vi "Control UI - Gain and Offset Exploration.vi"(9 "Active DUT index":i32 min=0 max=3 step=1, 10 "ESR scaling ref":refnum<vi>, 11 "Main Ref":refnum<class "Main.lvclass">) -> ()   [LabVIEW 2019, in "Main.lvclass"]
doc: "Developed by Kevin Thompson\nkevin@thompsonengineering.net\n\nCopyright 2020\nThompson Engineering, LLC"
uses:
  Main.lvclass
  support/Data Algorithms/subvis/DataTypes/ESR scaling--cluster.ctl
  Common/DataTypes/Inverter database record v2--cluster.ctl
  Common/DataTypes/inverter info v2--cluster.ctl
  Common/DataTypes/inverter gain range--cluster.ctl
  Common/DataTypes/inverter offset range--cluster.ctl
  Main.lvclass/Main.ctl
panel:
  in  "Direction":bool caption="Auto Increment Direction"
  in  "SetOffsetToMax":bool
  in  "SetGainToMax":bool
  in  "SetOffsetToMin":bool
  in  "SetGainToMin":bool
  in  "ResetGainOffsetRng":bool caption="Reset Gain/Offset\nRanges"
  in  "Exit":bool
  in  "Scaling Sel":enum32{"select gain", "select offset"}(radio) caption="Scaling Selection"
  in  "AutoIncrIntv (sec)":dbl(slide)=2.0 caption="Auto Increment Interval (sec)" min=2.0 max=20.0 step=1.0 scale=2.0..20.0
  out "AutoIncr LED":bool caption="Auto Incrementing"
  in  "StopAutoIncr":bool
  in  "StartAutoIncr":bool
  in  "offset range":T1
  in  "gain range":T2
  out "name":string caption="Inverter Name"
  out "CurrInverter":T3 {"last updated" format="%<%H:%M\n%d/%m/%Y>T"; "set flag" items=["False", "True"]}
  in  "StepBack":bool
  in  "StepFwd":bool
  in  "ESR scaling":T5={"Gain"=1.0, "Offset"=0.0} caption="Current ESR scaling" {"Offset" format="%^#_6g"; "Gain" format="%^#_6g"}
  # "Direction"
  # "increasing"
  # "decreasing"
  # "Inverter Gain & Offset Setting Explorer"
  # "Inverter Offset Range"
  # "Inverter Gain Range"
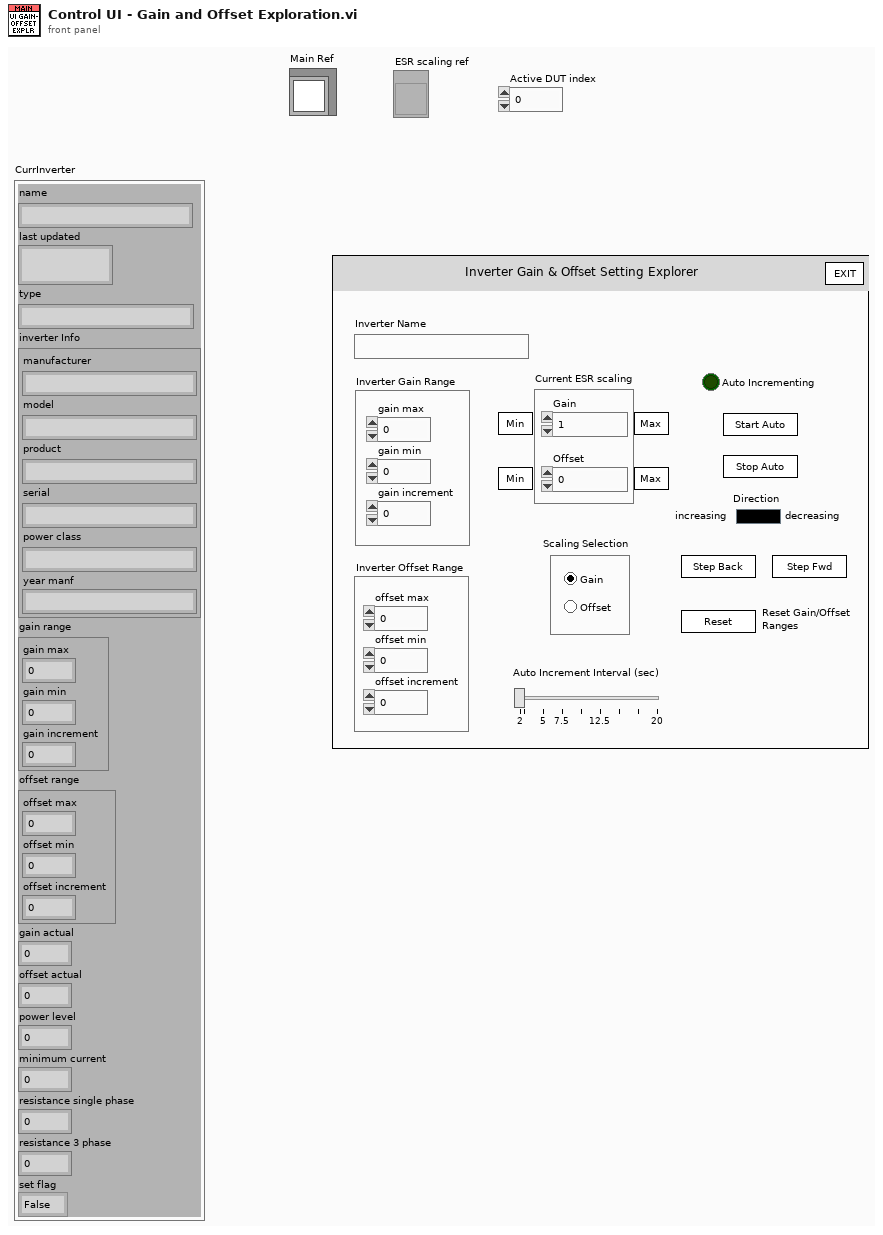
[diagram p1: front panel]
types:
  T1 = typedef "inverter offset range--cluster.ctl" = cluster{"offset max":dbl, "offset min":dbl, "offset increment":dbl}
  T2 = typedef "inverter gain range--cluster.ctl" = cluster{"gain max":dbl, "gain min":dbl, "gain increment":dbl}
  T3 = typedef "Inverter database record v2--cluster.ctl" = cluster{"name":string, "last updated":timestamp, "type":string, "inverter Info":T4, "gain range":T2, "offset range":T1, "gain actual":dbl, "offset actual":dbl, "power level":dbl, "minimum current":dbl, "resistance single phase":dbl, "resistance 3 phase":dbl, "set flag":u16}
  T4 = typedef "inverter info v2--cluster.ctl" = cluster{"manufacturer":string, "model":string, "product":string, "serial":string, "power class":string, "year manf":string}
  T5 = typedef "Main.lvclass/ESR scaling--cluster.ctl" = cluster{"Gain":dbl, "Offset":dbl}
  T6 = enum32{"invalid app kind", "Development System", "Run Time System", "Student Edition", "Embedded LabVIEW", "Evaluation", "Custom"}
  T7 = enum32{"Invalid", "Standard", "Closed", "Hidden", "Minimized", "Maximized"}
  T8 = cluster{"Main out":refnum<class "Main.lvclass">, "Core":cluster{"Current VI Reference":refnum<vi>, "Close Panel on Exit?":bool}, "ESR scaling ref":refnum<vi>, "ESR scaling":T5, "AutoIncr Enabled":bool, "Scaling Sel":enum32{"select gain", "select offset"}, "AutoIncrIntv (sec)":dbl, "ESR scaling - UI Label":string, "CurrInverter":T3, "gain range":T2, "offset range":T1, "Direction":bool, "LimitReached":bool}
  T9 = cluster{"Current VI Reference":refnum<vi>, "Close Panel on Exit?":bool}
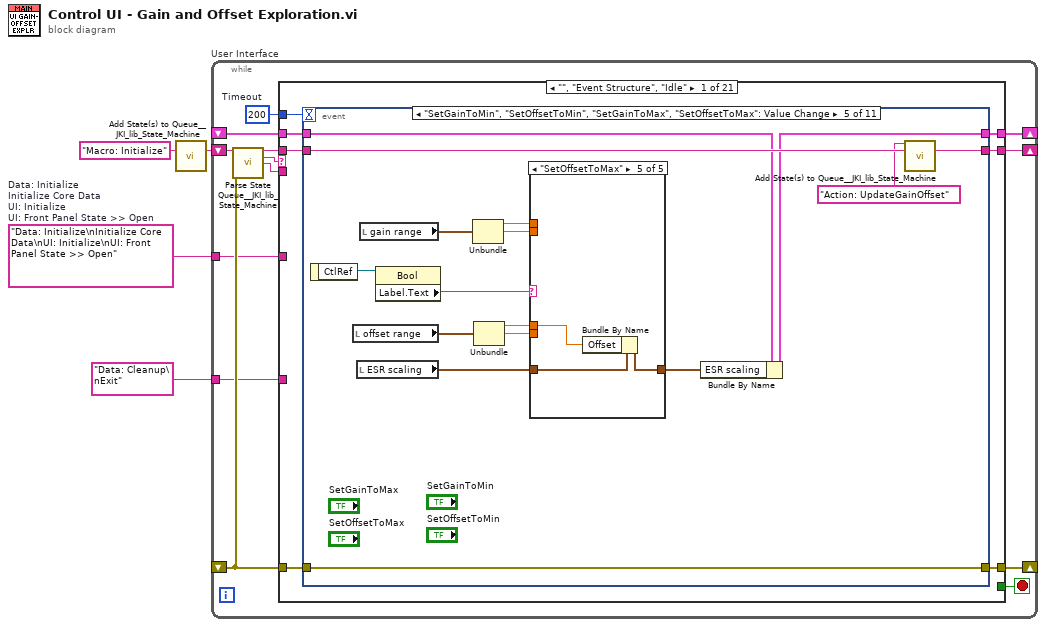
[diagram p0: block diagram]
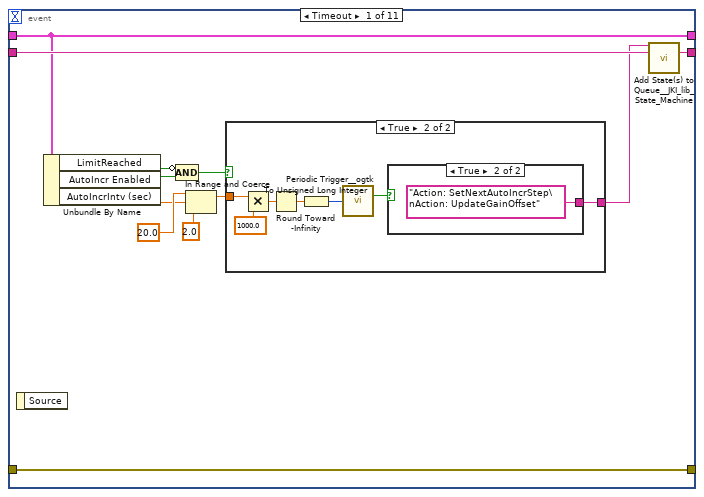
[diagram p2: hidden frame]
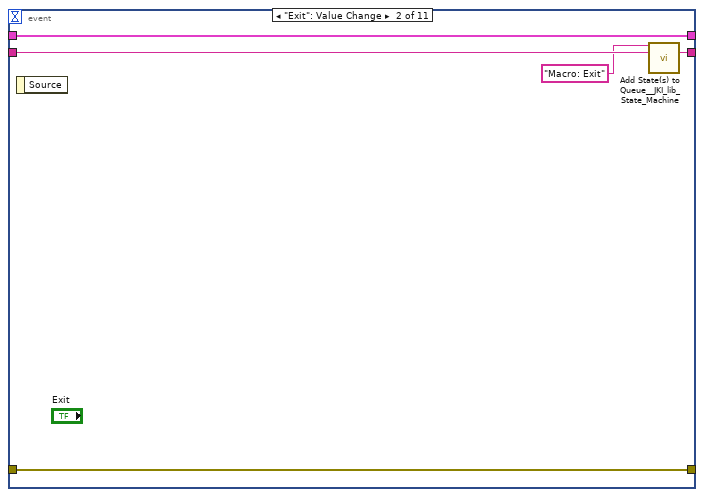
[diagram p5: hidden frame]
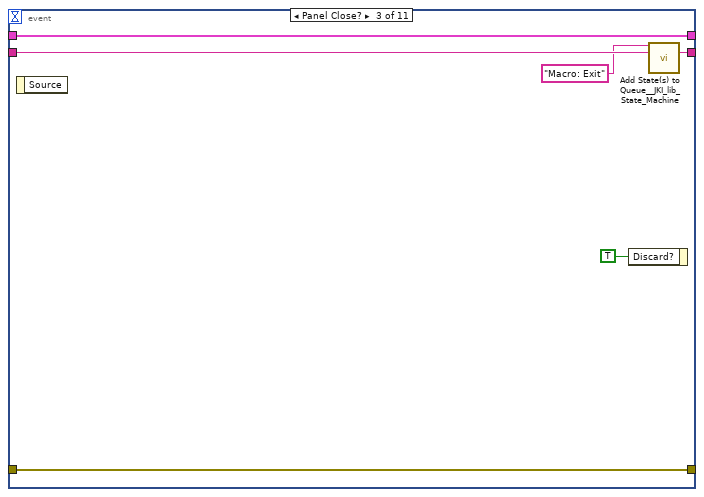
[diagram p6: hidden frame]
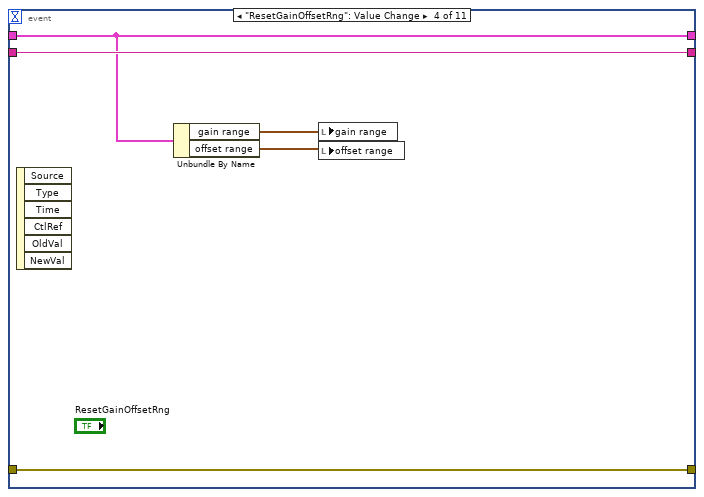
[diagram p7: hidden frame]
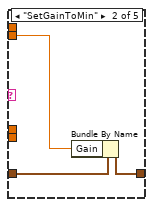
[diagram p9: hidden frame]
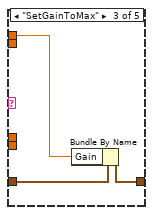
[diagram p10: hidden frame]
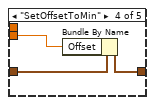
[diagram p11: hidden frame]
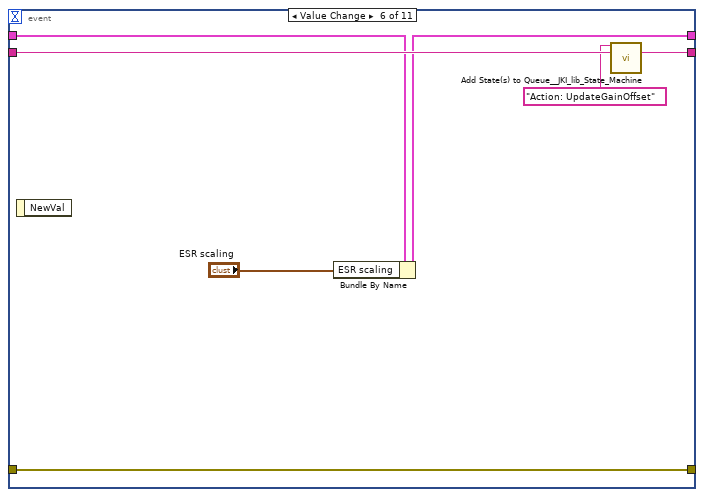
[diagram p12: hidden frame]
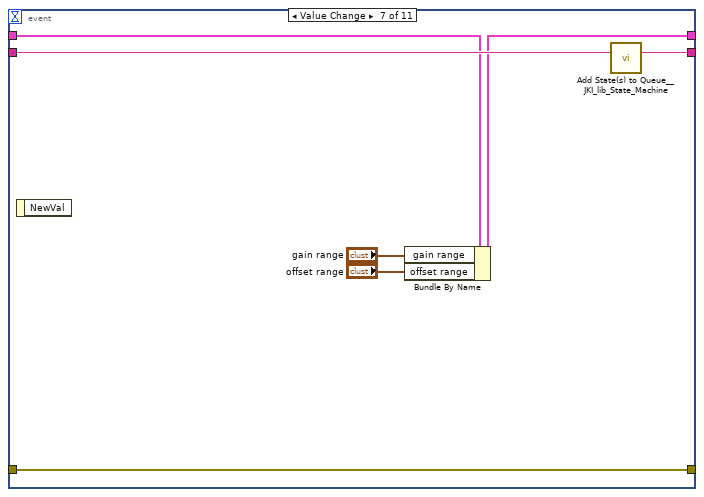
[diagram p13: hidden frame]
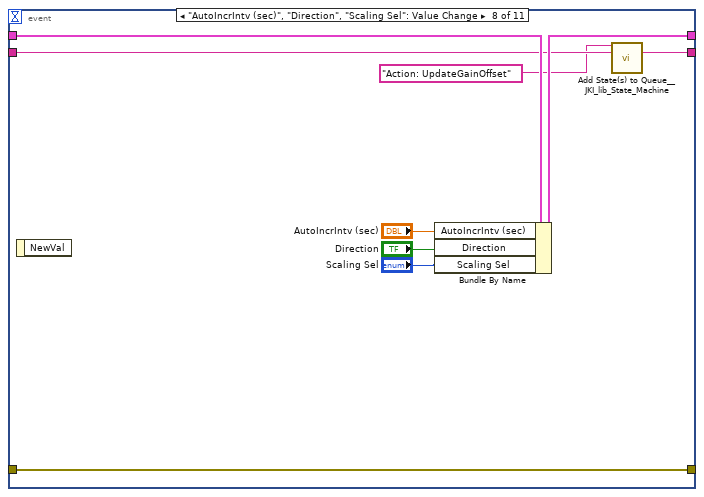
[diagram p14: hidden frame]
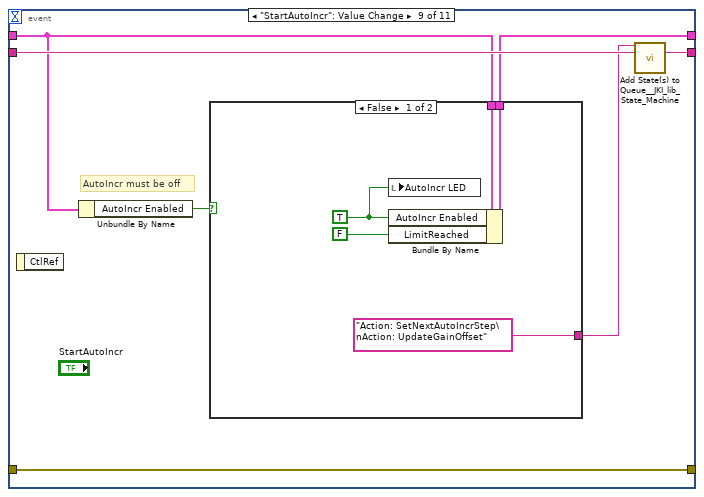
[diagram p15: hidden frame]
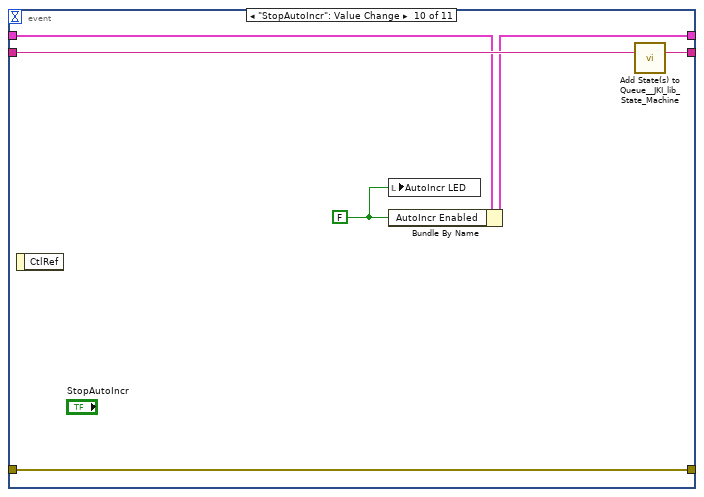
[diagram p17: hidden frame]
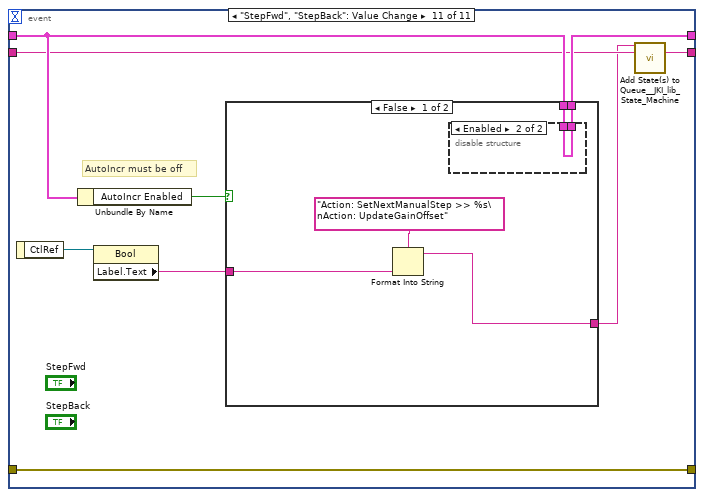
[diagram p18: hidden frame]
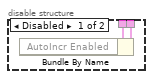
[diagram p19: hidden frame]
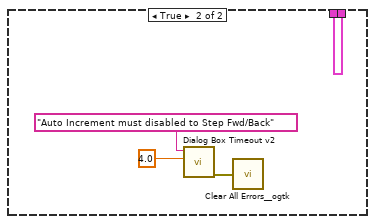
[diagram p20: hidden frame]
diagram:
  w2 = "Data: Initialize\nInitialize Core Data\nUI: Initialize\nUI: Front Panel State >> Open"  # Data: Initialize Initialize Core Data UI: Initialize UI: Front Panel State >> Open
  n1 = call <vilib>:"Add State(s) to Queue__JKI_lib_State_Machine.vi"("State(s) in (\"\")"="Macro: Initialize") -> ("States Out"=w4:string)  [unwired: 14 in]
  n2 = while "User Interface" {
    shift-right: [w10] -> _
    shift-left: _ -> [w9]
    shift-right: [w13] -> _
    shift-left: _ -> [w7]
    shift-right: [w12] -> _
    shift-left: w4 -> [w14]
    tunnel: w2 -> [w6]
    tunnel: "Data: Cleanup\nExit" -> [w5]
    stop <- w11 stop-if-true
    w8 = 200  # Timeout
    n3 = call <vilib>:"Parse State Queue__JKI_lib_State_Machine.vi"("State Queue"=w14, "Error In (no error)"=w7) -> ("Remaining States"=w16:string, "Current State"=w17:string, "Arguments"=w15:string)  [unwired: 11 in]
    n4 = case shown="\"\", \"Event Structure\", \"Idle\"" w17 {
      selector: w17 -> [_ _ w157 _ _ _ _ _ _ _ _ _ _ _ _ _ _ _ _ _ _]
      tunnel: w16 -> [w24 w156 w161 w179 w185 w190 w194 w221 w227 w231 w245 w252 w263 w289 w294 w304 w308 w315 w345 w405 w453]
      tunnel: w15 -> [_ _ _ _ _ _ _ _ _ _ _ w247 w257 _ _ _ _ _ w341 _ _]
      tunnel: w9 -> [w22 w153 w159 w170 w182 w188 w191 _ w222 w228 w240 w250 w259 w286 w291 w301 w305 w310 w324 w389 w450]
      tunnel: [w21 w154 w163 w176 errorcluster {"status"=FALSE, "code"=0, "source"=""} ("error out") w187 w192 w202 w223 w229 w243 w248 w260 w287 w292 w302 w306 w313 w343 w403 w447] -> w13
      tunnel: w7 -> [w20 w154 w162 w176 w181 w187 w192 w201 w224 w229 w243 w249 w261 w287 w292 w302 w306 w313 w343 w403 w446]
      tunnel: [w23 w155 w160 w178 w184 w189 w193 w220 w226 w230 w244 w251 w262 w288 w293 w303 w307 w314 w344 w404 w452] -> w12
      tunnel: [_ _ _ _ _ TRUE _ _ _ _ _ _ _ _ _ _ _ _ _ _ _] -> w11
      tunnel: [w19 w153 w159 w177 w182 w188 w191 w219 w222 w228 w241 w250 w259 w286 w291 w301 w305 w311 w325 w390 w450] -> w10
      tunnel: w8 -> [w18 _ _ _ _ _ _ _ _ _ _ _ _ _ _ _ _ _ _ _ _]
      tunnel: w6 -> [_ _ _ _ _ _ _ _ _ _ _ _ _ _ w290 _ _ _ _ _ _]
      tunnel: w5 -> [_ _ _ _ _ _ _ _ _ _ _ _ _ _ _ w295 _ _ _ _ _]
      frame "", "Event Structure", "Idle" {
        n5 = event shown="[4] \"SetGainToMin\", \"SetOffsetToMin\", \"SetGainToMax\", \"SetOffsetToMax\": Value Change" {
          selector: _ -> [_ _ _ _ _ _ _ _ _ _ _]
          dyn-events: _ -> [_ _ _ _ _ _ _ _ _ _ _]
          timeout: w18 -> [_ _ _ _ _ _ _ _ _ _ _]
          tunnel: w24 -> [w36 w49 w55 w60 w65 w94 w101 w105 w117 w129 w135]
          tunnel: [w35 w48 w54 w60 w66 w95 w102 w106 w118 w130 w136] -> w23
          tunnel: w22 -> [w33 w46 w52 w58 w61 w91 w99 w110 w113 w127 w137]
          tunnel: [w34 w47 w53 w59 w76 w96 w103 w112 w119 w131 w140] -> w21
          tunnel: w20 -> [w34 w47 w53 w59 w76 w96 w103 w112 w119 w131 w140]
          tunnel: [w33 w46 w52 w58 w62 w92 w100 w111 w115 w128 w138] -> w19
          event Timeout {
            n6 = event-data() -> ()  [unwired: 1 in, 1 out]
            n7 = Unbundle By Name(w33) -> ("LimitReached"=w25:bool, "AutoIncr Enabled"=w32:bool, "AutoIncrIntv (sec)"=w26:dbl)
            n8 = Compound Arithmetic op=AND(invert w25, w32) -> (w31:bool)
            n9 = In Range and Coerce(upper limit=20.0 ("lower limit"), x=w26, lower limit=2.0) -> (coerced(x)=w29:dbl)  [unwired: 1 out]
            n10 = case shown="True" w31 {
              tunnel: w29 -> [_ w40]
              tunnel: [_ w37] -> w30
              frame False {
              }
              frame True {
                n11 = Multiply(x=w40, y=1000.0) -> (x*y=w42:dbl)
                n12 = Round Toward -Infinity(1:w42) -> (0:w43:dbl)
                n13 = To Unsigned Long Integer(number=w43) -> (unsigned 32bit integer=w39:u32)
                n14 = call <userlib>:"Periodic Trigger__ogtk.vi"("time (ms)"=w39) -> ("Triggered"=w38:bool)  [unwired: 12 in, 2 out]
                n15 = case shown="True" w38 {
                  tunnel: [_ "Action: SetNextAutoIncrStep\nAction: UpdateGainOffset"] -> w37
                  frame False {
                  }
                  frame True {
                  }
                }
              }
            }
            n16 = call <vilib>:"Add State(s) to Queue__JKI_lib_State_Machine.vi"("State(s) in Front (\"\")"=w30, "State(s) in (\"\")"=w36) -> ("States Out"=w35:string)  [unwired: 13 in]
          }
          event "Exit": Value Change {
            n17 = event-data() -> ()  [unwired: 1 in, 1 out]
            n18 = call <vilib>:"Add State(s) to Queue__JKI_lib_State_Machine.vi"("State(s) in Front (\"\")"="Macro: Exit", "State(s) in (\"\")"=w49) -> ("States Out"=w48:string)  [unwired: 13 in]
          }
          event Panel Close? {
            n19 = event-data() -> ()  [unwired: 1 in, 1 out]
            n20 = event-data("Discard?"=TRUE) -> ()  [unwired: 1 in, 1 out]
            n21 = call <vilib>:"Add State(s) to Queue__JKI_lib_State_Machine.vi"("State(s) in Front (\"\")"="Macro: Exit", "State(s) in (\"\")"=w55) -> ("States Out"=w54:string)  [unwired: 13 in]
          }
          event "ResetGainOffsetRng": Value Change {
            n22 = event-data() -> ()  [unwired: 1 in, 6 out]
            n23 = Unbundle By Name(w58) -> ("gain range"=w57:T2, "offset range"=w56:T1)
            n24 = local write "gain range"(w57) -> ()
            n25 = local write "offset range"(w56) -> ()
          }
          event "SetGainToMin", "SetOffsetToMin", "SetGainToMax", "SetOffsetToMax": Value Change {
            n26 = event-data() -> ("CtlRef"=w75:refnum<vi>)  [unwired: 1 in]
            n27 = local read "offset range"() -> (w72:T1)
            n28 = local read "ESR scaling"() -> (w67:T5)
            n29 = local read "gain range"() -> (w73:T2)
            n30 = property class="Bool"(reference=w75) -> ("Label.Text"=w74:string)  [unwired: 1 in, 2 out]
            n31 = Unbundle(w73) -> ("gain max"=w71:dbl, "gain min"=w69:dbl)  [unwired: 1 out]
            n32 = Unbundle(w72) -> ("offset max"=w70:dbl, "offset min"=w68:dbl)  [unwired: 1 out]
            n33 = case shown="\"SetOffsetToMax\"" w74 {
              tunnel: w71 -> [_ _ w81 _ _]
              tunnel: w70 -> [_ _ _ _ w87]
              tunnel: w69 -> [_ w79 _ _ _]
              tunnel: w68 -> [_ _ _ w84 _]
              tunnel: w67 -> [w77 w80 w83 w86 w89]
              tunnel: [w77 w78 w82 w85 w88] -> w63
              frame Default {
              }
              frame "SetGainToMin" {
                n34 = Bundle By Name(cluster=w80, "Gain"=w79) -> (w78:T5)
              }
              frame "SetGainToMax" {
                n35 = Bundle By Name(cluster=w83, "Gain"=w81) -> (w82:T5)
              }
              frame "SetOffsetToMin" {
                n36 = Bundle By Name(cluster=w86, "Offset"=w84) -> (w85:T5)
              }
              frame "SetOffsetToMax" {
                n37 = Bundle By Name(cluster=w89, "Offset"=w87) -> (w88:T5)
              }
            }
            n38 = Bundle By Name(cluster=w61, "ESR scaling"=w63) -> (w62:T8)
            n39 = call <vilib>:"Add State(s) to Queue__JKI_lib_State_Machine.vi"("State(s) in Front (\"\")"="Action: UpdateGainOffset", "State(s) in (\"\")"=w65) -> ("States Out"=w66:string)  [unwired: 13 in]
          }
          event Value Change {
            n40 = event-data() -> ()  [unwired: 1 in, 1 out]
            n41 = Bundle By Name(cluster=w91, "ESR scaling"="ESR scaling") -> (w92:T8)
            n42 = call <vilib>:"Add State(s) to Queue__JKI_lib_State_Machine.vi"("State(s) in Front (\"\")"="Action: UpdateGainOffset", "State(s) in (\"\")"=w94) -> ("States Out"=w95:string)  [unwired: 13 in]
          }
          event Value Change {
            n43 = event-data() -> ()  [unwired: 1 in, 1 out]
            n44 = Bundle By Name(cluster=w99, "gain range"="gain range", "offset range"="offset range") -> (w100:T8)
            n45 = call <vilib>:"Add State(s) to Queue__JKI_lib_State_Machine.vi"("State(s) in (\"\")"=w101) -> ("States Out"=w102:string)  [unwired: 14 in]
          }
          event "AutoIncrIntv (sec)", "Direction", "Scaling Sel": Value Change {
            n46 = event-data() -> ()  [unwired: 1 in, 1 out]
            n47 = Bundle By Name(cluster=w110, "AutoIncrIntv (sec)"="AutoIncrIntv (sec)", "Direction"="Direction", "Scaling Sel"="Scaling Sel") -> (w111:T8)
            n48 = call <vilib>:"Add State(s) to Queue__JKI_lib_State_Machine.vi"("State(s) in Front (\"\")"="Action: UpdateGainOffset", "State(s) in (\"\")"=w105) -> ("States Out"=w106:string)  [unwired: 13 in]
          }
          event "StartAutoIncr": Value Change {
            # "AutoIncr must be off"
            n49 = event-data() -> ()  [unwired: 1 in, 1 out]
            n50 = Unbundle By Name(w113) -> ("AutoIncr Enabled"=w116:bool)
            n51 = case shown="False" w116 {
              tunnel: w113 -> [w124 w125]
              tunnel: [w123 w125] -> w115
              tunnel: ["Action: SetNextAutoIncrStep\nAction: UpdateGainOffset" _] -> w114
              frame False {
                w120 = TRUE ("AutoIncr Enabled")
                n52 = local write "AutoIncr LED"(w120) -> ()
                n53 = Bundle By Name(cluster=w124, "AutoIncr Enabled"=w120, "LimitReached"=FALSE) -> (w123:T8)
              }
              frame True {
              }
            }
            n54 = call <vilib>:"Add State(s) to Queue__JKI_lib_State_Machine.vi"("State(s) in Front (\"\")"=w114, "State(s) in (\"\")"=w117) -> ("States Out"=w118:string)  [unwired: 13 in]
          }
          event "StopAutoIncr": Value Change {
            w126 = FALSE ("AutoIncr Enabled")
            n55 = event-data() -> ()  [unwired: 1 in, 1 out]
            n56 = local write "AutoIncr LED"(w126) -> ()
            n57 = Bundle By Name(cluster=w127, "AutoIncr Enabled"=w126) -> (w128:T8)
            n58 = call <vilib>:"Add State(s) to Queue__JKI_lib_State_Machine.vi"("State(s) in (\"\")"=w129) -> ("States Out"=w130:string)  [unwired: 14 in]
          }
          event "StepFwd", "StepBack": Value Change {
            # "AutoIncr must be off"
            n59 = event-data() -> ("CtlRef"=w133:refnum<vi>)  [unwired: 1 in]
            n60 = Unbundle By Name(w137) -> ("AutoIncr Enabled"=w139:bool)
            n61 = property class="Bool"(reference=w133) -> ("Label.Text"=w132:string)  [unwired: 1 in, 2 out]
            n62 = case shown="False" w139 {
              tunnel: w137 -> [w145 w152]
              tunnel: [w144 w152] -> w138
              tunnel: [w141 _] -> w134
              tunnel: w132 -> [w142 _]
              frame False {
                n63 = Format Into String(format string="Action: SetNextManualStep >> %s\nAction: UpdateGainOffset", w142) -> (resulting string=w141:string)  [unwired: 2 in, 1 out]
                n64 = disable-structure shown="Enabled" {
                  disable-tunnel: w145 -> [w147 w148]
                  disable-tunnel: [w146 w148] -> w144
                  frame Disabled {
                    n65 = Bundle By Name(cluster=w147) -> (w146:T8)  [unwired: 1 in]
                  }
                  frame Enabled {
                  }
                }
              }
              frame True {
                n66 = call "Dialog Box Timeout v2.vi"("Timeout (s)"=4.0, "Message"="Auto Increment must disabled to Step Fwd/Back") -> ("Error Out"=w149:errorcluster)  [unwired: 9 in]
                n67 = call <userlib>:"Clear All Errors__ogtk.vi"("Error In"=w149) -> ()  [unwired: 3 in, 1 out]
              }
            }
            n68 = call <vilib>:"Add State(s) to Queue__JKI_lib_State_Machine.vi"("State(s) in Front (\"\")"=w134, "State(s) in (\"\")"=w135) -> ("States Out"=w136:string)  [unwired: 13 in]
          }
        }
      }
      frame "---------- Core ----------" {
        n69 = call <vilib>:"Add State(s) to Queue__JKI_lib_State_Machine.vi"("State(s) in (\"\")"=w156) -> ("States Out"=w155:string)  [unwired: 14 in]
      }
      frame Default {
        w166 = 42 items=["No error", "Argument error", "Memory is full", "Out of zone", "End of file", "File already open", "Generic file I/O error", "File not found", "File permission error", "Disk is full", "Duplicate path", "Too many files open", "System feature not enabled", "Resource file not found", "Cannot add resource", "Resource not found", "Image not found", "Image memory error", "Pen does not exist", "Config type invalid", "Config token not found", "Config parse error", "Config memory error", "Bad external code format", "Bad external code offset", "External code not present", "Null window", "Destroy window error", "Null menu", "Print aborted", "Bad print record", "Print driver error", "Windows error during printing", "Memory error during printing", "Print dialog error", "Generic print error", "Invalid device refnum", "Device not found", "Device parameter error", "Device unit error", "Cannot open device", "Device call aborted", "Generic error", "Cancelled by user", "Object ID too low", "Object ID too high", "Object not in heap", "Unknown heap", "Unknown object (invalid DefProc)", "Unknown object (DefProc not in table)", "Message out of range", "Invalid (null) method", "Unknown message", "Manager call not supported", "Bad address", "Network operation in progress", "Network operation timed out", "Connection is busy", "Network attribute not supported", "Network error", "Address in use", "System out of memory", "Connection aborted", "Connection refused", "Not connected", "Already connected", "Connection closed", "Initialization error (interapplication manager)", "Bad occurrence", "Wait on unbound occurrence handler", "Occurrence queue overflow", "Datalog type conflict", "Unused", "Unrecognized type (interapplication manager)", "Memory corrupt", "Failed to make temporary DLL", "Old CIN version", "Drag socket not found", "Failed to load drop-object", "Failed to register OLE object", "Failed to release OLE object", "Format specifier type mismatch", "Unknown format specifier", "Too few format specifiers", "Too many format specifiers", "Scan failed", "Newer CIN version", "Error converting to variant", "Runtime menu error", "Password tampered", "Variant attribute not found", "Incompatible variant data type", "Event data is not available", "Event Store is not present", "Occurrence is not found", "Event Queue is not created", "Event info is not available", "Refnum passed is NULL", "Error retrieving Class GUID", "Error retrieving CoClass GUID", "Error retrieving TypeLib GUID.", "Bad built application magic bytes.", "Specific driver is different from the specific driver associated with the Logical Name.", "There is no session opened to the class driver.", "Max Error", "MAX - Error with config objects", "MAX - Error loading configuration", "MAX - Group not supported"]
        # "Current State"
        n70 = Format Into String(format string="Software Exception: Unhandled State \"%s\"." ("message"), error in=w162, w157) -> (resulting string=w165:string, error out=w164:errorcluster)  [unwired: 1 in]
        n71 = call <vilib>:"Error Cluster From Error Code.vi"("show call chain? (False)"=TRUE, "error in (no error)"=w164, "error message (\"\")"=w165, "error code (0)"=w166) -> ("error out"=w163:errorcluster)  [unwired: 5 in]
        n72 = call <vilib>:"Add State(s) to Queue__JKI_lib_State_Machine.vi"("State(s) in (\"\")"=w161) -> ("States Out"=w160:string)  [unwired: 14 in]
      }
      frame "Initialize Core Data" {
        # "originally closed?"
        # "exe?"
        n73 = property class="VI"() -> ("Front Panel.Open"=w175:bool)  [unwired: 2 in, 2 out]
        n74 = property class="App"() -> ("App.Kind"=w174:T6)  [unwired: 2 in, 2 out]
        n75 = control-ref of="Current VI Reference"() -> (w168:refnum<vi>)
        n76 = Not(x=w175) -> (.not. x?=w172:bool)
        n77 = Equal?(x=w174, y=T6."Run Time System" ("Application:Kind")) -> (x = y?=w171:bool)
        n78 = Or(x=w172, y=w171) -> (x .or. y?=w169:bool)
        n79 = Bundle By Name(cluster=w170, "Core.Current VI Reference"=w168, "Core.Close Panel on Exit?"=w169) -> (w177:T8)
        n80 = call <vilib>:"Add State(s) to Queue__JKI_lib_State_Machine.vi"("State(s) in (\"\")"=w179) -> ("States Out"=w178:string)  [unwired: 14 in]
      }
      frame "Error Handler" {
        n81 = call <vilib>:"General Error Handler.vi"("error in (no error)"=w181) -> ()  [unwired: 10 in, 5 out]
        n82 = call <vilib>:"Add State(s) to Queue__JKI_lib_State_Machine.vi"("State(s) in Front (\"\")"="/* Post Error States", "State(s) in (\"\")"=w185) -> ("States Out"=w184:string)  [unwired: 13 in]
      }
      frame "Exit" {
        n83 = call <vilib>:"Add State(s) to Queue__JKI_lib_State_Machine.vi"("State(s) in (\"\")"=w190) -> ("States Out"=w189:string)  [unwired: 14 in]
      }
      frame "---------- Data ----------" {
        n84 = call <vilib>:"Add State(s) to Queue__JKI_lib_State_Machine.vi"("State(s) in (\"\")"=w194) -> ("States Out"=w193:string)  [unwired: 14 in]
      }
      frame "Data: Initialize" {
        w207 = FALSE  # LimitReached
        w208 = FALSE  # Direction
        (unwired) T1 {"offset max"=0.0, "offset min"=0.0, "offset increment"=0.0}  # offset range
        (unwired) T2 {"gain max"=0.0, "gain min"=0.0, "gain increment"=0.0}  # gain range
        w211 = T5 {"Gain"=0.0, "Offset"=0.0}  # ESR scaling
        w215 = "ESR scaling"  # ESR scaling - UI Label
        w216 = 5.0  # AutoIncrIntv (sec)
        w217 = enum32{"select gain", "select offset"}."select gain"  # Scaling Sel
        w218 = FALSE  # AutoIncr Enabled
        w212 = T9 {"Current VI Reference"=refnum, "Close Panel on Exit?"=FALSE}  # Core
        n85 = call "Get CurrInverter Record.vi"("error in (no error)"=w201, "Main in"="Main Ref") -> ("error out"=w203:errorcluster, "CurrInverters"=w204:T3[], "Main out"=w205:refnum<class "Main.lvclass">)  [unwired: 7 in]
        n86 = property class="Arr (strict)"(reference="ESR scaling ref", error in=w203) -> (reference out=w213:refnum<vi>, error out=w209:errorcluster, "Value"=w200:T5[])
        n87 = Index Array(array=w204, index="Active DUT index") -> (element=w197:T3)
        "CurrInverter" <- w197
        n88 = Unbundle By Name(w197) -> ("gain range"=w196:T2, "offset range"=w195:T1)
        n89 = Index Array(array=w200, index="Active DUT index") -> (element=w198:T5)
        n90 = Variant To Data(error in=w209, type=w211, Variant=w198) -> (data=w210:T5, error out=w202:errorcluster)
        n91 = local write "ESR scaling"(w210) -> ()
        n92 = call <vilib>:"Add State(s) to Queue__JKI_lib_State_Machine.vi"("State(s) in (\"\")"=w221) -> ("States Out"=w220:string)  [unwired: 14 in]
        n93 = Bundle("Main out"=w205, "Core"=w212, "ESR scaling ref"=w213, "ESR scaling"=w210, "AutoIncr Enabled"=w218, "Scaling Sel"=w217, "AutoIncrIntv (sec)"=w216, "ESR scaling - UI Label"=w215, "CurrInverter"=w197, "gain range"=w196, "offset range"=w195, "Direction"=w208, "LimitReached"=w207) -> (w219:T8)  [unwired: 1 in]
      }
      frame "Data: Cleanup" {
        n94 = Unbundle By Name(w222) -> ("Core.Current VI Reference"=w225:refnum<vi>)
        n95 = Close Reference(reference=w225, error in (no error)=w224) -> (error out=w223:errorcluster)
        n96 = call <vilib>:"Add State(s) to Queue__JKI_lib_State_Machine.vi"("State(s) in (\"\")"=w227) -> ("States Out"=w226:string)  [unwired: 14 in]
      }
      frame "---------- UI ----------" {
        n97 = call <vilib>:"Add State(s) to Queue__JKI_lib_State_Machine.vi"("State(s) in (\"\")"=w231) -> ("States Out"=w230:string)  [unwired: 14 in]
      }
      frame "UI: Initialize" {
        n98 = Unbundle By Name(w240) -> ("CurrInverter.name"=→"name":string, "gain range"=w238:T2, "offset range"=w239:T1, "Core.Current VI Reference"=w233:refnum<vi>)
        n99 = call <userlib>:"Fit VI window to Largest Dec__ogtk.vi"("VI Ref (calling VI)"=w233) -> ("dup VI Ref"=w232:refnum<vi>)  [unwired: 5 in, 1 out]
        n100 = disable-structure shown="Disabled" {
          disable-tunnel: w232 -> [w246 _]
          frame Disabled {
            n101 = property class="VI" props=["Front Panel.Title"](reference=w246) -> ()  [unwired: 2 in, 2 out]
          }
          frame Enabled {
          }
        }
        n102 = local write "gain range"(w238) -> ()
        n103 = local write "offset range"(w239) -> ()
        n104 = Bundle By Name(cluster=w240, "gain range"=w238, "offset range"=w239) -> (w241:T8)
        n105 = local write "Scaling Sel"(enum32{"select gain", "select offset"}."select gain" ("AutoIncr Sel")) -> ()
        n106 = local write "AutoIncrIntv (sec)"(5.0 ("AutoIncrIntv (sec)")) -> ()
        n107 = local write "Direction"(FALSE) -> ()
        n108 = call <vilib>:"Add State(s) to Queue__JKI_lib_State_Machine.vi"("State(s) in (\"\")"=w245) -> ("States Out"=w244:string)  [unwired: 14 in]
        "AutoIncr LED" <- FALSE
      }
      frame "UI: Cursor Set" {
        # "Argument"
        n109 = case shown="\"Idle\", Default" w247 {
          tunnel: w249 -> [w254 w256]
          tunnel: [w253 w255] -> w248
          frame "Idle", Default {
            n110 = call <vilib>:"Unset Busy.vi"("error in (no error)"=w254) -> ("error out"=w253:errorcluster)  [unwired: 10 in]
          }
          frame "Busy" {
            n111 = call <vilib>:"Set Busy.vi"("error in (no error)"=w256) -> ("error out"=w255:errorcluster)  [unwired: 9 in, 1 out]
          }
        }
        n112 = call <vilib>:"Add State(s) to Queue__JKI_lib_State_Machine.vi"("State(s) in (\"\")"=w252) -> ("States Out"=w251:string)  [unwired: 14 in]
      }
      frame "UI: Front Panel State" {
        # "Argument"
        n113 = Unbundle By Name(w259) -> ("Core.Current VI Reference"=w258:refnum<vi>)
        n114 = case shown="\"Open\", Default" w257 {
          tunnel: w261 -> [w267 w280]
          tunnel: [w269 w281] -> w260
          tunnel: w258 -> [w268 w278]
          frame "Open", Default {
            n115 = property class="VI"(reference=w268, error in=w267) -> (reference out=w265:refnum<vi>, error out=w266:errorcluster, "Front Panel.Open"=w264:bool)
            n116 = case shown="False" w264 {
              tunnel: [w272 w275] -> w269
              tunnel: w266 -> [w271 w275]
              tunnel: w265 -> [w270 _]
              frame False {
                n117 = invoke class="VI" method="FP.Open"(reference=w270, error in=w271, "Activate"=TRUE, "State"=T7."Standard") -> (error out=w272:errorcluster)  [unwired: 1 in, 4 out]
              }
              frame True {
              }
            }
          }
          frame "Close" {
            n118 = property class="VI"(reference=w278, error in=w280) -> (reference out=w277:refnum<vi>, error out=w279:errorcluster, "Front Panel.Open"=w276:bool)
            n119 = case shown="True" w276 {
              tunnel: [w282 w285] -> w281
              tunnel: w279 -> [w282 w284]
              tunnel: w277 -> [_ w283]
              frame False {
              }
              frame True {
                n120 = invoke class="VI" method="FP.Close"(reference=w283, error in=w284) -> (error out=w285:errorcluster)  [unwired: 1 in, 2 out]
              }
            }
          }
        }
        n121 = call <vilib>:"Add State(s) to Queue__JKI_lib_State_Machine.vi"("State(s) in (\"\")"=w263) -> ("States Out"=w262:string)  [unwired: 14 in]
      }
      frame "---------- Macro ----------" {
        n122 = call <vilib>:"Add State(s) to Queue__JKI_lib_State_Machine.vi"("State(s) in (\"\")"=w289) -> ("States Out"=w288:string)  [unwired: 14 in]
      }
      frame "Macro: Initialize" {
        n123 = call <vilib>:"Add State(s) to Queue__JKI_lib_State_Machine.vi"("State(s) in Front (\"\")"=w290, "State(s) in (\"\")"=w294) -> ("States Out"=w293:string)  [unwired: 13 in]
      }
      frame "Macro: Exit" {
        n124 = Unbundle By Name(w301) -> ("Core.Close Panel on Exit?"=w300:bool)
        n125 = Select(t="UI: Front Panel State >> Close", s=w300, f="") -> (s? t:f=w297:string)
        n126 = call <vilib>:"Add State(s) to Queue__JKI_lib_State_Machine.vi"("State(s) in (\"\")"=w297, "State(s) at Back (\"\")"=w295) -> ("States Out"=w296:string)  [unwired: 13 in]
        n127 = call <vilib>:"Add State(s) to Queue__JKI_lib_State_Machine.vi"("State(s) in Front (\"\")"=w296, "State(s) in (\"\")"=w304) -> ("States Out"=w303:string)  [unwired: 13 in]
      }
      frame "---------- Action ----------" {
        n128 = call <vilib>:"Add State(s) to Queue__JKI_lib_State_Machine.vi"("State(s) in (\"\")"=w308) -> ("States Out"=w307:string)  [unwired: 14 in]
      }
      frame "Action: Reset AutoIncrEnable" {
        w312 = FALSE ("AutoIncr Enabled")
        n129 = One Button Dialog(message="Max/Min Limit reached.") -> ()  [unwired: 1 in, 1 out]
        n130 = local write "AutoIncr LED"(w312) -> ()
        n131 = Bundle By Name(cluster=w310, "AutoIncr Enabled"=w312) -> (w311:T8)
        n132 = call <vilib>:"Add State(s) to Queue__JKI_lib_State_Machine.vi"("State(s) in (\"\")"=w315) -> ("States Out"=w314:string)  [unwired: 14 in]
      }
      frame "Action: SetNextManualStep" {
        n133 = Unbundle By Name(w324) -> ("Scaling Sel"=w323:enum32{"select gain", "select offset"}, "ESR scaling.Gain"=w331:dbl, "ESR scaling.Offset"=w330:dbl, "gain range.gain max"=w340:dbl, "gain range.gain min"=w339:dbl, "gain range.gain increment"=w338:dbl, "offset range.offset max"=w337:dbl, "offset range.offset min"=w336:dbl, "offset range.offset increment"=w335:dbl)
        n134 = Unbundle By Name(w324) -> ("Direction"=w333:bool)
        n135 = Equal?(x=w341, y="StepFwd") -> (x = y?=w334:bool)
        n136 = case shown="\"select gain\", Default" w323 {
          tunnel: w340 -> [w373 _]
          tunnel: w339 -> [w372 _]
          tunnel: w338 -> [w371 _]
          tunnel: w337 -> [_ w379]
          tunnel: w336 -> [_ w378]
          tunnel: w335 -> [_ w377]
          tunnel: [w373 w379] -> w328
          tunnel: [w372 w378] -> w327
          tunnel: [w371 w377] -> w326
          tunnel: w331 -> [w374 w375]
          tunnel: w330 -> [w370 w376]
          tunnel: [w374 w376] -> w329
          tunnel: [w370 w375] -> w320
          frame "select gain", Default {
          }
          frame "select offset" {
          }
        }
        n137 = Compound Arithmetic op=XOR(w333, w334) -> (w332:bool)
        n138 = case shown="False" w332 {
          tunnel: w329 -> [w362 w369]
          tunnel: w328 -> [w357 w364]
          tunnel: w327 -> [w358 w365]
          tunnel: w326 -> [w361 w368]
          tunnel: [w360 w367] -> w321
          tunnel: [w356 w363] -> w322
          frame True {
            n139 = Add(x=w362, y=w361) -> (x+y=w359:dbl)
            n140 = In Range and Coerce(upper limit=w357, x=w359, lower limit=w358) -> (coerced(x)=w360:dbl, In Range?=w356:bool)
          }
          frame False {
            n141 = Subtract(x=w369, y=w368) -> (x-y=w366:dbl)
            n142 = In Range and Coerce(upper limit=w364, x=w366, lower limit=w365) -> (coerced(x)=w367:dbl, In Range?=w363:bool)
          }
        }
        n143 = Not(x=w322) -> (.not. x?=w316:bool)
        n144 = case shown="\"select gain\", Default" w323 {
          tunnel: [w350 w355] -> w325
          tunnel: w324 -> [w349 w354]
          tunnel: w316 -> [w348 w353]
          tunnel: w321 -> [w347 w352]
          tunnel: w320 -> [w346 w351]
          frame "select gain", Default {
            n145 = Bundle By Name(cluster=w349, "ESR scaling.Offset"=w346, "ESR scaling.Gain"=w347, "LimitReached"=w348) -> (w350:T8)
          }
          frame "select offset" {
            n146 = Bundle By Name(cluster=w354, "ESR scaling.Gain"=w351, "ESR scaling.Offset"=w352, "LimitReached"=w353) -> (w355:T8)
          }
        }
        n147 = Select(t="Action: Reset AutoIncrEnable", s=w316, f="") -> (s? t:f=w317:string)
        n148 = call <vilib>:"Add State(s) to Queue__JKI_lib_State_Machine.vi"("State(s) in Front (\"\")"=w317, "State(s) in (\"\")"=w345) -> ("States Out"=w344:string)  [unwired: 13 in]
      }
      frame "Action: SetNextAutoIncrStep" {
        n149 = Unbundle By Name(w389) -> ("Scaling Sel"=w388:enum32{"select gain", "select offset"}, "ESR scaling.Gain"=w396:dbl, "ESR scaling.Offset"=w395:dbl, "gain range.gain max"=w402:dbl, "gain range.gain min"=w401:dbl, "gain range.gain increment"=w400:dbl, "offset range.offset max"=w399:dbl, "offset range.offset min"=w398:dbl, "offset range.offset increment"=w397:dbl)
        n150 = Unbundle By Name(w389) -> ("Direction"=w384:bool)
        n151 = case shown="\"select offset\"" w388 {
          tunnel: w402 -> [w433 _]
          tunnel: w401 -> [w432 _]
          tunnel: w400 -> [w431 _]
          tunnel: w399 -> [_ w439]
          tunnel: w398 -> [_ w438]
          tunnel: w397 -> [_ w437]
          tunnel: [w433 w439] -> w393
          tunnel: [w432 w438] -> w392
          tunnel: [w431 w437] -> w391
          tunnel: w396 -> [w434 w435]
          tunnel: w395 -> [w430 w436]
          tunnel: [w434 w436] -> w394
          tunnel: [w430 w435] -> w385
          frame "select gain", Default {
          }
          frame "select offset" {
          }
        }
        n152 = case shown="False" w384 {
          tunnel: w394 -> [w422 w429]
          tunnel: w393 -> [w417 w424]
          tunnel: w392 -> [w418 w425]
          tunnel: w391 -> [w421 w428]
          tunnel: [w420 w427] -> w386
          tunnel: [w416 w423] -> w387
          frame True {
            n153 = Subtract(x=w422, y=w421) -> (x-y=w419:dbl)
            n154 = In Range and Coerce(upper limit=w417, x=w419, lower limit=w418) -> (coerced(x)=w420:dbl, In Range?=w416:bool)
          }
          frame False {
            n155 = Add(x=w429, y=w428) -> (x+y=w426:dbl)
            n156 = In Range and Coerce(upper limit=w424, x=w426, lower limit=w425) -> (coerced(x)=w427:dbl, In Range?=w423:bool)
          }
        }
        n157 = Not(x=w387) -> (.not. x?=w380:bool)
        n158 = case shown="\"select offset\"" w388 {
          tunnel: [w410 w415] -> w390
          tunnel: w389 -> [w409 w414]
          tunnel: w380 -> [w406 w411]
          tunnel: w386 -> [w408 w413]
          tunnel: w385 -> [w407 w412]
          frame "select gain", Default {
            n159 = Bundle By Name(cluster=w409, "ESR scaling.Offset"=w407, "ESR scaling.Gain"=w408, "LimitReached"=w406) -> (w410:T8)
          }
          frame "select offset" {
            n160 = Bundle By Name(cluster=w414, "ESR scaling.Gain"=w412, "ESR scaling.Offset"=w413, "LimitReached"=w411) -> (w415:T8)
          }
        }
        n161 = Select(t="Action: Reset AutoIncrEnable", s=w380, f="") -> (s? t:f=w381:string)
        n162 = call <vilib>:"Add State(s) to Queue__JKI_lib_State_Machine.vi"("State(s) in Front (\"\")"=w381, "State(s) in (\"\")"=w405) -> ("States Out"=w404:string)  [unwired: 13 in]
      }
      frame "Action: UpdateGainOffset" {
        # "update local control"
        # "Update Main process"
        # "update Main UI"
        n163 = Unbundle By Name(w450) -> ("ESR scaling - UI Label"=w449:string, "Main out"=w451:refnum<class "Main.lvclass">, "ESR scaling"=w443:T5, "ESR scaling ref"=w441:refnum<vi>)
        n164 = property class="Arr (strict)"(reference=w441) -> (reference out=w440:refnum<vi>, "Value"=w445:T5[])  [unwired: 1 in, 1 out]
        n165 = local read "Active DUT index"() -> (w444:i32)
        n166 = local write "ESR scaling"(w443) -> ()
        n167 = Replace Array Subset(array=w445, new element=w443, index=w444) -> (w442:T5[])
        n168 = property class="Arr (strict)"(reference=w440, error in=w446, "Value"=w442) -> (error out=w448:errorcluster)  [unwired: 1 out]
        n169 = call "Fire UpdateControlValue Event.vi"("error in (no error)"=w448, "vData"=w442, "Control Label"=w449, "Main in"=w451) -> ("error out"=w447:errorcluster)  [unwired: 6 in, 1 out]
        n170 = call <vilib>:"Add State(s) to Queue__JKI_lib_State_Machine.vi"("State(s) in (\"\")"=w453) -> ("States Out"=w452:string)  [unwired: 14 in]
      }
    }
  }
